vi "Dir Checker.vi"(11 "System Data":T1={"System"={"Active"=FALSE, "Exit"=FALSE, "Command wait"="", "Status_Time"=0, "Time_GPS"=0}, "Stepper Motor"={"Connection Reference"="", "Valid Connection"=FALSE, "Speed"=15}, "Camera Data"={"Image path"=path "", "Filenames"=[], "Filenames queue"=[]}, "Core"={"Close Panel on Exit?"=FALSE, "Current VI Reference"=refnum}} {"Stepper Motor"."Speed" scale=0.0..30.0}) -> (0 "error constant":errorcluster, 1 "Image path":path, 3 "System Data Out":T1={"System"={"Active"=FALSE, "Exit"=FALSE, "Command wait"="", "Status_Time"=0, "Time_GPS"=0}, "Stepper Motor"={"Connection Reference"="", "Valid Connection"=FALSE, "Speed"=15}, "Camera Data"={"Image path"=path "", "Filenames"=[], "Filenames queue"=[]}, "Core"={"Close Panel on Exit?"=FALSE, "Current VI Reference"=refnum}} {"Stepper Motor"."Speed" scale=0.0..30.0})   [LabVIEW 2019]
uses:
  System Data.ctl
  Stepper Data.ctl
  Camera Data.ctl
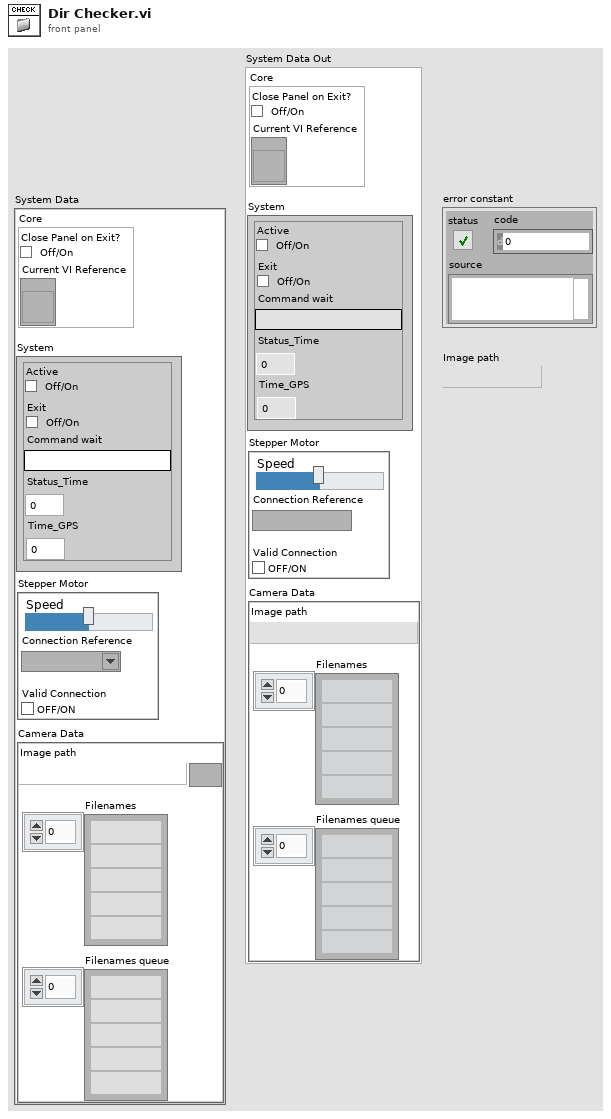
[diagram p1: front panel]
types:
  T1 = typedef "System Data.ctl" = cluster{"System":cluster{"Active":bool, "Exit":bool, "Command wait":string, "Status_Time":i32, "Time_GPS":i32}, "Stepper Motor":T2, "Camera Data":T3, "Core":cluster{"Close Panel on Exit?":bool, "Current VI Reference":refnum<vi>}}
  T2 = typedef "Stepper Data.ctl" = cluster{"Connection Reference":refnum<visa-resource-name>, "Valid Connection":bool, "Speed":i32}
  T3 = typedef "Camera Data.ctl" = cluster{"Image path":path, "Filenames":string[], "Filenames queue":string[]}
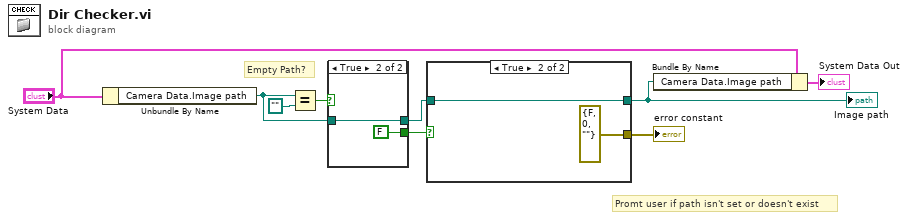
[diagram p0: block diagram]
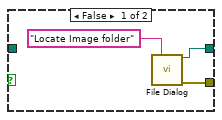
[diagram p2: hidden frame]
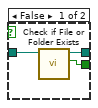
[diagram p3: hidden frame]
diagram:
  # "Promt user if path isn't set or doesn't exist"
  # "Empty Path?"
  n1 = Unbundle By Name("System Data") -> ("Camera Data.Image path"=w2:path)
  n2 = Equal?(x=w2, y=path "") -> (x = y?=w8:bool)
  n3 = case shown="True" w8 {
    tunnel: w2 -> [w12 w13]
    tunnel: [w11 FALSE ("file or folder exists?")] -> w7
    tunnel: [w10 w13] -> w5
    frame False {
      n4 = call <vilib>:"Check if File or Folder Exists.vi"("path"=w12) -> ("file or folder exists?"=w11:bool, "dup path"=w10:path)  [unwired: 8 in, 1 out]
    }
    frame True {
    }
  }
  n5 = case shown="True" w7 {
    tunnel: [w16 w19] -> w3
    tunnel: w5 -> [_ w19]
    tunnel: [w15 errorcluster {"status"=FALSE, "code"=0, "source"=""} ("error constant")] -> w1
    frame False {
      n6 = call "File Dialog"("prompt"="Locate Image folder") -> ("selected path"=w16:path, "error out"=w15:errorcluster)  [unwired: 11 in, 2 out]
    }
    frame True {
    }
  }
  "error constant" <- w1
  "Image path" <- w3
  n7 = Bundle By Name(cluster="System Data", "Camera Data.Image path"=w3) -> (→"System Data Out":T1)
